vi "ReadAndParseXML.vi"() -> (2 "XML Elements":string[](array[string]))   [LabVIEW 2009, in "NavScreen.lvlib"]
uses:
  NavScreen.lvlib
panel:
  out "error out":errorcluster
  in  "error in (no error)":errorcluster
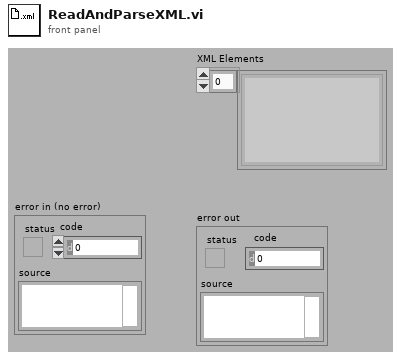
[diagram p1: front panel]
types:
  T1 = enum16{"open", "replace", "create", "open or create", "replace or create", "replace or create with confirmation"}
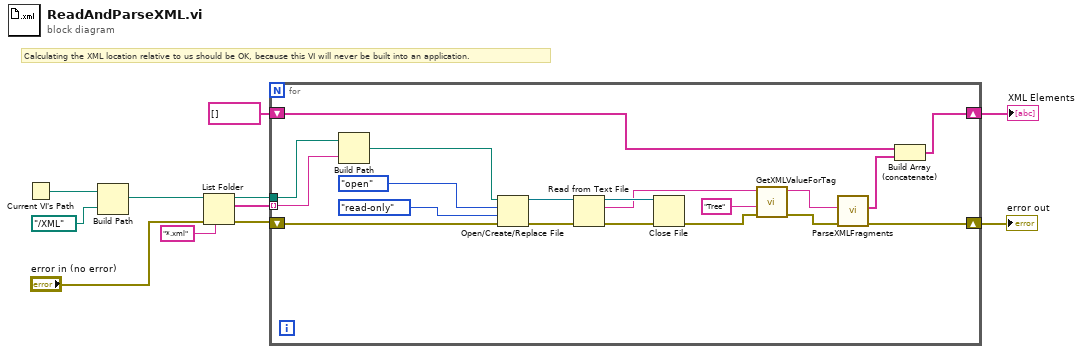
[diagram p0: block diagram]
diagram:
  # "Calculating the XML location relative to us should be OK, because this VI will never be built into an application."
  n1 = Current VI's Path() -> (path=w3:path)
  n2 = Build Path(base path=w3, name or relative path=path "../XML") -> (appended path=w10:path)
  n3 = List Folder(path=w10, pattern="*.xml", error in="error in (no error)") -> (path out=w5:path, filenames=w7:string[], error out=w9:errorcluster)  [unwired: 1 in, 1 out]
  n4 = for {
    shift-right: [w29] -> w11
    shift-left: w9 -> [w20]
    tunnel: w7 -> [w18] mode=indexing
    tunnel: w5 -> [w19]
    shift-right: [w12] -> w4
    shift-left: string[] [] -> [w13]
    n5 = Build Path(base path=w19, name or relative path=w18) -> (appended path=w17:path)
    n6 = Open/Create/Replace File(file path (use dialog)=w17, error in=w20, operation (0:open)=T1."open", access (0:read/write)=enum16{"read/write", "read-only", "write-only"}."read-only") -> (refnum out=w24:refnum<file>, error out=w25:errorcluster)  [unwired: 2 in, 1 out]
    n7 = Read from Text File(file (use dialog)=w24, error in=w25) -> (refnum out=w30:refnum<file>, text=w23:string, error out=w28:errorcluster)  [unwired: 2 in, 1 out]
    n8 = Close File(refnum=w30, error in=w28) -> (error out=w16:errorcluster)  [unwired: 1 out]
    n9 = call "GetXMLValueForTag.vi"("error in (no error)"=w16, "tag"="Tree", "XML"=w23) -> ("error out"=w15:errorcluster, "value"=w22:string)  [unwired: 7 in]
    n10 = call <vilib>:"ParseXMLFragments.vi"("error in (no error)"=w15, "XML in"=w22) -> ("error out"=w29:errorcluster, "XML Elements"=w14:string[])  [unwired: 8 in]
    n11 = Build Array (concatenate)(w13, w14) -> (w12:string[])
  }
  "error out" <- w11
  "XML Elements" <- w4
